vi "数据查询_仪器日志.vi"() -> ()   [LabVIEW 2016]
uses:
  <vilib>/Utility/miscctls.llb/LVRowAndColumnUnsignedTypeDef.ctl
  <vilib>/Utility/miscctls.llb/LVPointTypeDef.ctl
  <userlib>/_OpenG.lib/array/array.llb/Remove Duplicates from 1D Array (String)__ogtk.vi
panel:
  in  "查询":bool
  out "数据表":string[][](table)
  in  "结束日期":string="2020/01/01"
  in  "起始日期":string="2010/01/01"
  in  "组合框":string(combo)
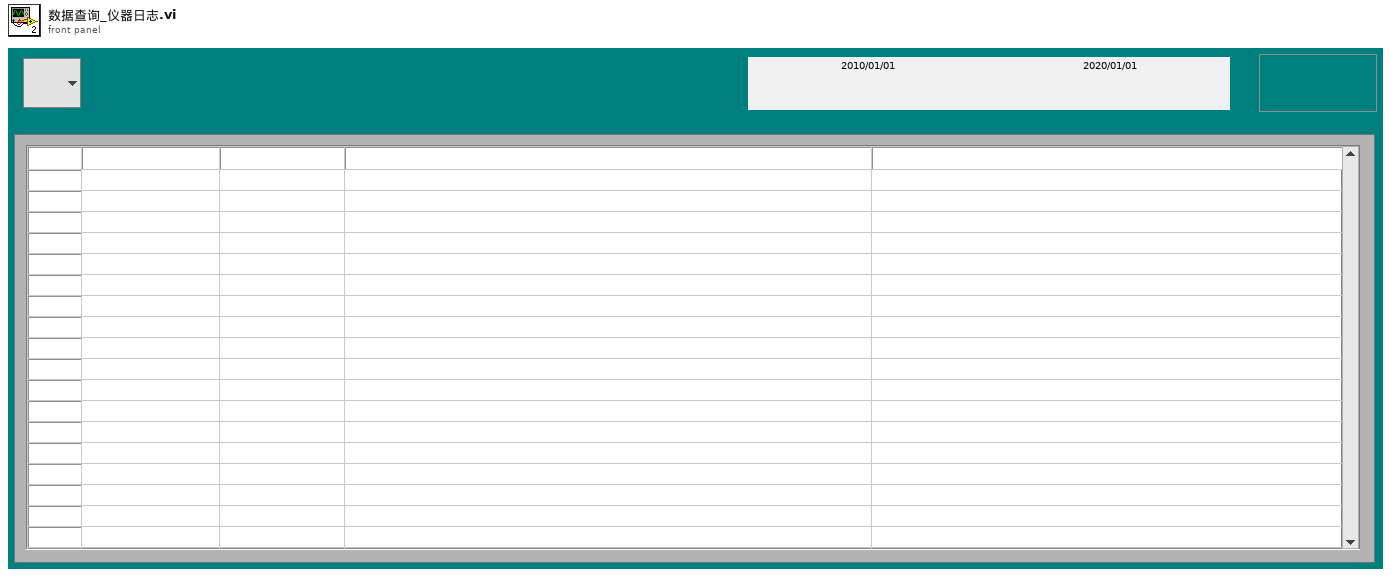
[diagram p1: front panel]
types:
  T1 = typedef "LVRowAndColumnUnsignedTypeDef.ctl" = cluster{"Row":u32, "Column":u32}
  T2 = typedef "LVPointTypeDef.ctl" = cluster{"Horizontal":i16, "Vertical":i16}
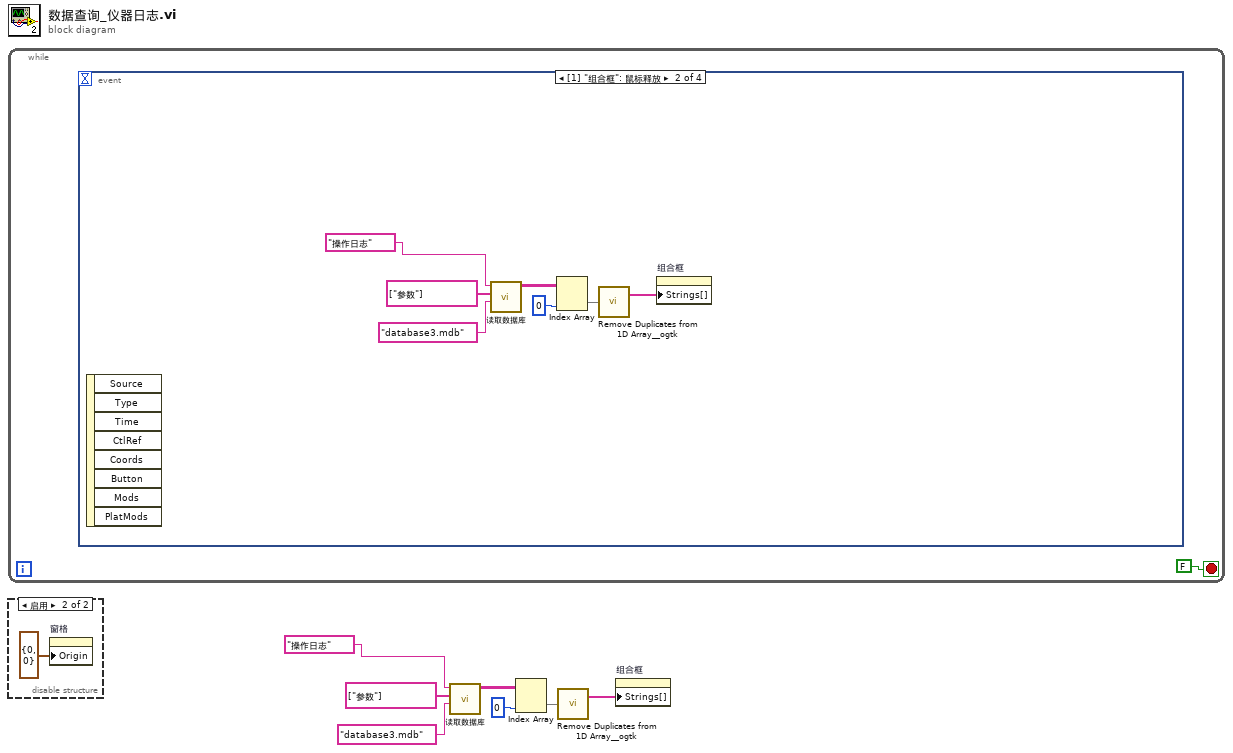
[diagram p0: block diagram]
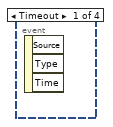
[diagram p2: hidden frame]
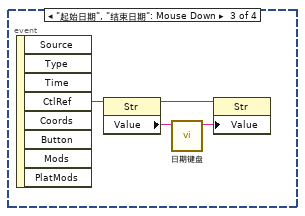
[diagram p3: hidden frame]
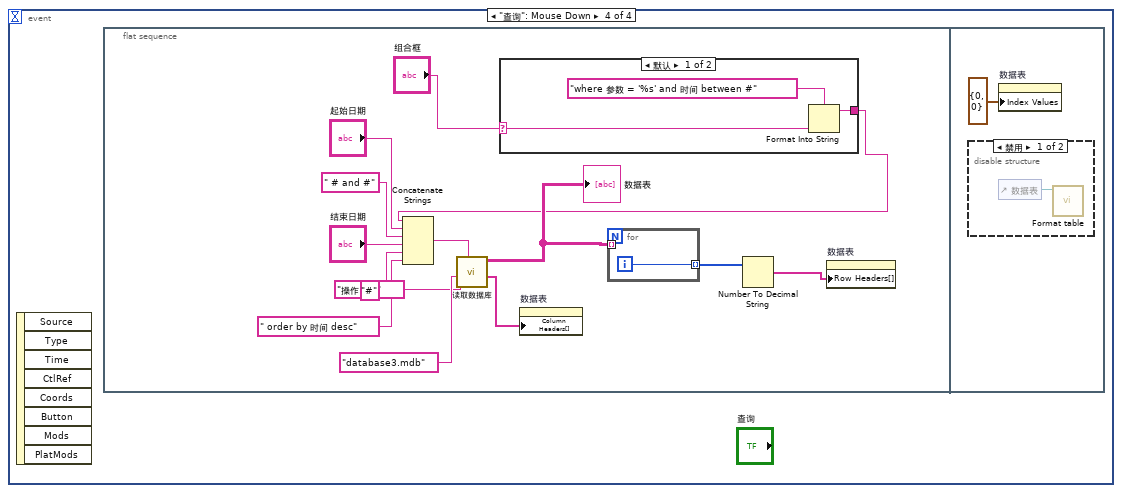
[diagram p4: hidden frame]
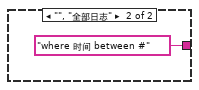
[diagram p5: hidden frame]
diagram:
  n1 = while {
    stop <- FALSE stop-if-true
    n2 = event shown="[1] \"组合框\": 鼠标释放" {
      selector: _ -> [_ _ _ _]
      dyn-events: _ -> [_ _ _ _]
      timeout: _ -> [_ _ _ _]
      event Timeout {
        n3 = event-data() -> ()  [unwired: 1 in, 3 out]
      }
      event "组合框": Mouse Up {
        n4 = event-data() -> ()  [unwired: 1 in, 8 out]
        n5 = call "读取数据库.vi"("database"="database3.mdb", "显示项"=string[] ["参数"], "组合框"="操作日志") -> ("表格"=w11:string[][])  [unwired: 5 in, 3 out]
        n6 = Index Array(array=w11, index (col)=0 ("禁用的索引 (列)")) -> (element=w12:string[])  [unwired: 1 in]
        n7 = call-poly <userlib>:"Remove Duplicates from 1D Array__ogtk.vi"("Input Array"=w12) -> ("Output Array"=w14:string[])  [unwired: 1 out]
        n8 = property on="组合框" class="CmbBox"("Strings[]"=w14) -> ()  [unwired: 2 in, 2 out]
      }
      event "起始日期", "结束日期": Mouse Down {
        n9 = event-data() -> ("CtlRef"=w19:refnum<vi>)  [unwired: 1 in, 7 out]
        n10 = property class="Str"(reference=w19) -> (reference out=w17:refnum<vi>, "Value"=w18:string)  [unwired: 1 in, 1 out]
        n11 = call "日期键盘.vi"("原值"=w18) -> ("x+y"=w16:string)  [unwired: 10 in]
        n12 = property class="Str"(reference=w17, "Value"=w16) -> ()  [unwired: 1 in, 2 out]
      }
      event "查询": Mouse Down {
        n13 = event-data() -> ()  [unwired: 1 in, 8 out]
        n14 = flat-sequence {
          frame #0 {
            n15 = case shown="默认" "组合框" {
              selector: "组合框" -> [w34 _]
              tunnel: [w36 "where 时间 between #" ("condition")] -> w20
              frame Default {
                n16 = Format Into String(format string="where 参数 = '%s' and 时间 between #" ("condition"), w34) -> (resulting string=w36:string)  [unwired: 2 in, 1 out]
              }
              frame "", "全部日志" {
              }
            }
            n17 = Concatenate Strings(w20, "起始日期", " # and #" ("condition"), "结束日期", "#" ("condition"), " order by 时间 desc" ("字符串")) -> (w32:string)
            n18 = call "读取数据库.vi"("condition"=w32, "database"="database3.mdb", "组合框"="操作日志") -> ("columns"=w28:string[], "表格"=w25:string[][])  [unwired: 5 in, 2 out]
            "数据表" <- w25
            n19 = property on="数据表" class="Tbl (严格)"("Column Headers[]"=w28) -> ()  [unwired: 2 in, 2 out]
            n20 = for {
              tunnel: w25 -> [_] mode=indexing
              tunnel: [w38] -> w24 mode=indexing
              i -> [w38]
            }
            n21 = Number To Decimal String(number=w24) -> (decimal integer string=w23:string[])  [unwired: 1 in]
            n22 = property on="数据表" class="Tbl (严格)"("Row Headers[]"=w23) -> ()  [unwired: 2 in, 2 out]
          }
          frame #1 {
            n23 = disable-structure shown="禁用" {
              frame Disabled {
                n24 = control-ref of="数据表"() -> (w40:refnum<vi>)
                n25 = call "Format table.vi"("Table输入"=w40) -> ()  [unwired: 11 in]
              }
              frame Enabled {
              }
            }
            n26 = property on="数据表" class="Tbl (严格)"("Index Values"=T1 {"Row"=0, "Column"=0} ("索引值")) -> ()  [unwired: 2 in, 2 out]
          }
        }
      }
    }
  }
  n27 = disable-structure shown="启用" {
    frame Disabled {
    }
    frame Enabled {
      n28 = property on="窗格" class="Pane"("Origin"=T2 {"Horizontal"=0, "Vertical"=0} ("原点")) -> ()  [unwired: 2 in, 2 out]
    }
  }
  n29 = call "读取数据库.vi"("database"="database3.mdb", "显示项"=string[] ["参数"], "组合框"="操作日志") -> ("表格"=w5:string[][])  [unwired: 5 in, 3 out]
  n30 = Index Array(array=w5, index (col)=0 ("禁用的索引 (列)")) -> (element=w4:string[])  [unwired: 1 in]
  n31 = call-poly <userlib>:"Remove Duplicates from 1D Array__ogtk.vi"("Input Array"=w4) -> ("Output Array"=w2:string[])  [unwired: 1 out]
  n32 = property on="组合框" class="CmbBox"("Strings[]"=w2) -> ()  [unwired: 2 in, 2 out]
